vi "Single Channel Temperature Log with Header.vi"() -> ()   [LabVIEW 2014]
doc: "本VI每间隔1秒采集温度值。本VI也计算最近5次温度测量值的平均值，并通过波形图表显示原始数据和实时平均值。本VI将原始数据保存至文本文件中。"
panel:
  in  "停止按钮":bool
  out "温度历史":cluster{dbl, "Temperature Value":dbl}(graph)
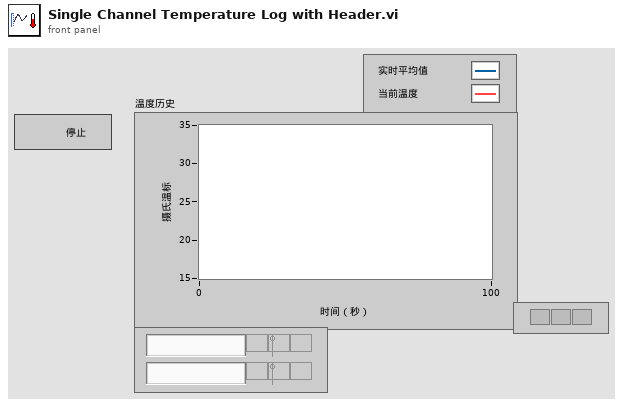
[diagram p1: front panel]
types:
  T1 = enum16{"open", "replace", "create", "open or create", "replace or create", "replace or create with confirmation"}
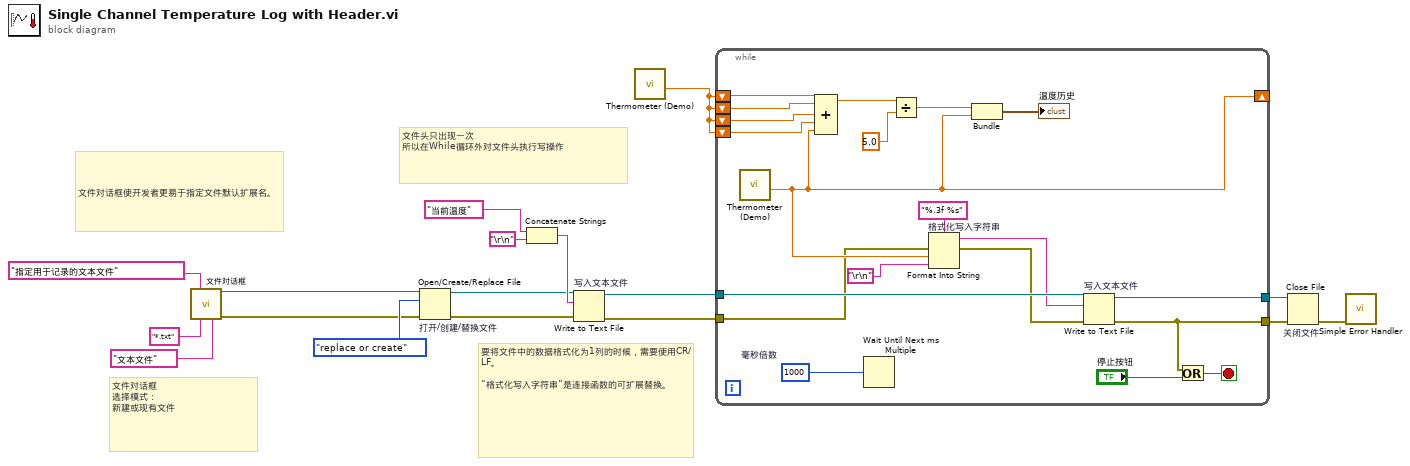
[diagram p0: block diagram]
diagram:
  # "文件对话框\n选择模式：\n新建或现有文件"
  # "要将文件中的数据格式化为1列的时候，需要使用CR/LF。\n\n“格式化写入字符串”是连接函数的可扩展替换。"
  # "文件头只出现一次\n所以在While循环外对文件头执行写操作"
  # "文件对话框使开发者更易于指定文件默认扩展名。"
  n1 = call "文件对话框"("prompt"="指定用于记录的文本文件" ("类型标签"), "pattern (all files)"="*.txt" ("类型（所有文件）"), "pattern label"="文本文件" ("类型标签")) -> ("selected path"=w7:path, "error out"=w1:errorcluster)  [unwired: 9 in, 2 out]
  n2 = Open/Create/Replace File "打开/创建/替换文件"(file path (use dialog)=w7, error in=w1, operation (0:open)=T1."replace or create" ("操作(0:open)")) -> (refnum out=w10:refnum<file>, error out=w11:errorcluster)  [unwired: 4 out]
  n3 = Concatenate Strings("当前温度" ("字符串"), "\r\n" ("行结束常量")) -> (w12:string)
  n4 = Write to Text File "写入文本文件"(file (use dialog)=w10, text=w12, error in=w11) -> (refnum out=w4:refnum<file>, error out=w3:errorcluster)  [unwired: 2 out]
  n5 = call "Thermometer (Demo).vi"() -> ("温度值"=w17:dbl)  [unwired: 11 in]
  n6 = while {
    shift-right: [w23] -> _
    shift-left: w17 -> [w36]
    shift-left: w17 -> [w35]
    shift-left: w17 -> [w32]
    shift-left: w17 -> [w31]
    tunnel: w3 -> [w21]
    tunnel: [w26] -> w15
    tunnel: w4 -> [w28]
    tunnel: [w27] -> w14
    stop <- w24 stop-if-true
    w37 = u32 1000  # 毫秒倍数
    n7 = call "Thermometer (Demo).vi"() -> ("温度值"=w23:dbl)  [unwired: 11 in]
    n8 = Compound Arithmetic op=ADD(w36, w35, w32, w31, w23) -> (w34:dbl)
    n9 = Wait Until Next ms Multiple(millisecond multiple=w37) -> ()  [unwired: 1 out]
    n10 = Divide(x=w34, y=5.0) -> (x/y=w30:dbl)
    n11 = Format Into String "格式化写入字符串"(format string="%.3f %s" ("格式字符串"), error in=w21, w23, "\r\n" ("行结束常量")) -> (resulting string=w22:string, error out=w20:errorcluster)  [unwired: 1 in]
    n12 = Bundle(w30, "温度值"=w23) -> (→"温度历史":cluster{dbl, "温度值":dbl})  [unwired: 1 in]
    n13 = Write to Text File "写入文本文件"(file (use dialog)=w28, text=w22, error in=w20) -> (refnum out=w27:refnum<file>, error out=w26:errorcluster)  [unwired: 2 out]
    n14 = Or(x=w26, y="停止按钮") -> (x .or. y?=w24:bool)
  }
  n15 = Close File "关闭文件"(refnum=w14, error in=w15) -> (error out=w16:errorcluster)  [unwired: 1 out]
  n16 = call <vilib>:"Simple Error Handler.vi"("error in (no error)"=w16) -> ()  [unwired: 1 in, 8 out]
